vi "GoalVisionCalibrationHelper.vi"(8 "HSV Filter":refnum<vi>, 10 "Src Image":T1, 11 "Image Ctl Refnum":refnum<vi>) -> ()   [LabVIEW 2013]
uses:
  <vilib>/vision/Image Controls.llb/IMAQ Image.ctl
panel:
  in  "Std Devs":cluster{"Hue":dbl, "Sat":dbl, "Val":dbl}={"Hue"=4.0, "Sat"=6.0, "Val"=4.0}
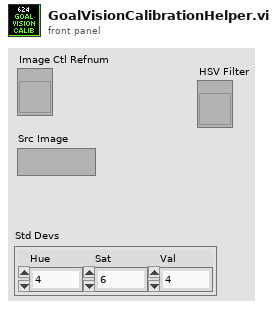
[diagram p1: front panel]
types:
  T1 = typedef "IMAQ Image.ctl" = refnum<image>
  T2 = cluster{"Hue":cluster{dbl, dbl}, "Sat":cluster{dbl, dbl}, "Val":cluster{dbl, dbl}}
  T3 = cluster{"Hue min":dbl, "Hue max":dbl, "Sat min":dbl, "Sat max":dbl, "Lum min":dbl, "Lum max":dbl}
  T4 = cluster{cluster{dbl, dbl}, cluster{dbl, dbl}, cluster{dbl, dbl}}
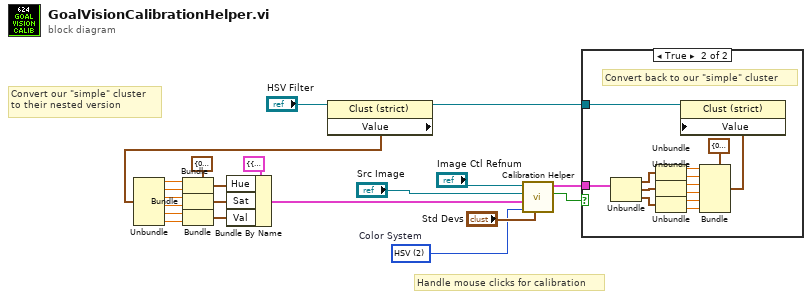
[diagram p0: block diagram]
diagram:
  w2 = u16 2 items=["RGB", "HSL", "HSV", "HSI"]  # Color System
  w16 = cluster{dbl, dbl} {0.0, 0.0} ("Hue")
  # "Convert our \"simple\" cluster\nto their nested version"
  # "Handle mouse clicks for calibration"
  n1 = property class="Clust (strict)"(reference="HSV Filter") -> (reference out=w3:refnum<vi>, "Value"=w5:T3)  [unwired: 1 in, 1 out]
  n2 = Unbundle(w5) -> ("Hue min"=w13:dbl, "Hue max"=w12:dbl, "Sat min"=w11:dbl, "Sat max"=w10:dbl, "Lum min"=w9:dbl, "Lum max"=w8:dbl)
  n3 = Bundle(cluster=w16, w13, w12) -> (w17:cluster{dbl, dbl})
  n4 = Bundle(cluster=w16, w11, w10) -> (w15:cluster{dbl, dbl})
  n5 = Bundle(cluster=w16, w9, w8) -> (w14:cluster{dbl, dbl})
  n6 = Bundle By Name(cluster=T2 {"Hue"={104.99307782068851, 142.0}, "Sat"={138.0, 255.0}, "Val"={139.0, 198.0}} ("Color Components"), "Hue"=w17, "Sat"=w15, "Val"=w14) -> (w4:T2)
  n7 = call "Calibration Helper.vi"("Std Devs"="Std Devs", "Color Mode"=w2, "Color Components"=w4, "Image"="Src Image", "Image Ctl Refnum"="Image Ctl Refnum") -> ("Changed"=w19:bool, "output color"=w20:T4)  [unwired: 5 in]
  n8 = case shown="True" w19 {
    tunnel: w20 -> [_ w23]
    tunnel: w3 -> [_ w34]
    frame False {
    }
    frame True {
      # "Convert back to our \"simple\" cluster"
      n9 = Unbundle(w23) -> (w24:cluster{dbl, dbl}, w25:cluster{dbl, dbl}, w26:cluster{dbl, dbl})
      n10 = Unbundle(w24) -> (w28:dbl, w29:dbl)
      n11 = Unbundle(w25) -> (w30:dbl, w31:dbl)
      n12 = Unbundle(w26) -> (w32:dbl, w33:dbl)
      n13 = Bundle(cluster=T3 {"Hue min"=0.0, "Hue max"=0.0, "Sat min"=0.0, "Sat max"=0.0, "Lum min"=0.0, "Lum max"=0.0} ("HSV Filter 2"), "Hue min"=w28, "Hue max"=w29, "Sat min"=w30, "Sat max"=w31, "Lum min"=w32, "Lum max"=w33) -> (w22:T3)
      n14 = property class="Clust (strict)"(reference=w34, "Value"=w22) -> ()  [unwired: 1 in, 2 out]
    }
  }
